vi "Open SubPanel.vi"() -> ()   [LabVIEW 2021]
panel:
  out "error out":errorcluster
  in  "error in":errorcluster
  in  "Stop Button":bool
  in  "Select VI":i32(ring) items=["Show Time", "Random Numbers", "Sine Wave"]
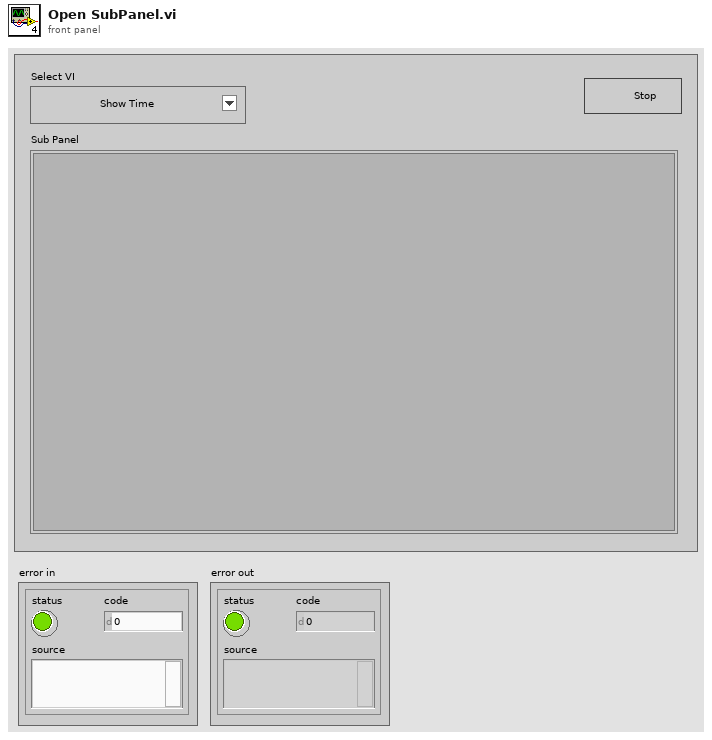
[diagram p1: front panel]
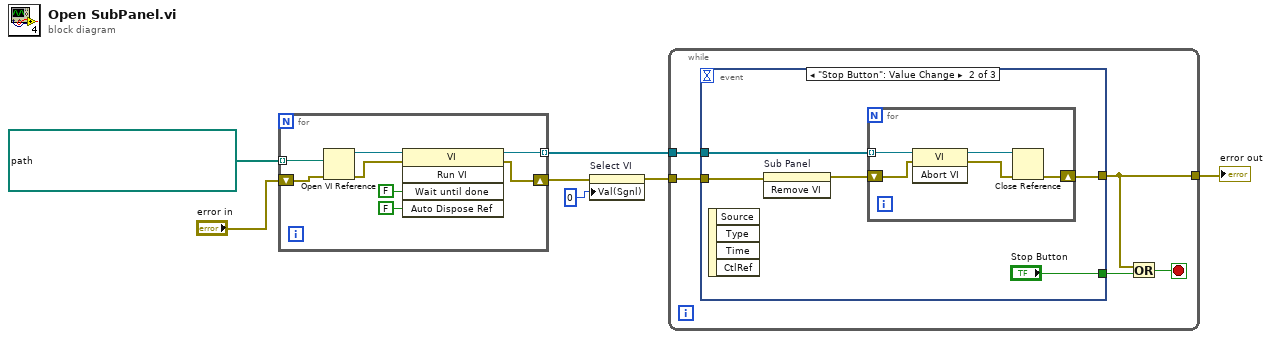
[diagram p0: block diagram]
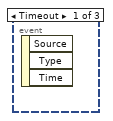
[diagram p2: hidden frame]
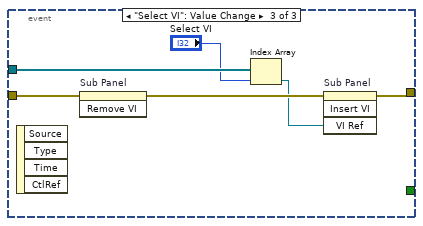
[diagram p3: hidden frame]
diagram:
  n1 = for {
    tunnel: path[] [path "F:/AGH - Inżynieria Biomedyczna (I i II stopień)/PRACA MAGISTERSKA/LABVIEW - examples (CODE)/Using SubPanels/Demo - Current Time.vi", path "F:/AGH - Inżynieria Biomedyczna (I i II stopień)/PRACA MAGISTERSKA/LABVIEW - examples (CODE)/Using SubPanels/Demo - Random Data Chart.vi", path "F:/AGH - Inżynieria Biomedyczna (I i II stopień)/PRACA MAGISTERSKA/LABVIEW - examples (CODE)/Using SubPanels/Demo - Sine Graph.vi"] -> [w15] mode=indexing
    shift-right: [w9] -> w4
    shift-left: "error in" -> [w14]
    tunnel: [w8] -> w5 mode=indexing
    n2 = Open VI Reference(vi path=w15, error in (no error)=w14) -> (vi reference=w11:refnum<vi>, error out=w10:errorcluster)  [unwired: 4 in]
    n3 = invoke class="VI" method="Run VI"(reference=w11, error in=w10, "Wait until done"=FALSE ("Wait Until Done"), "Auto Dispose Ref"=FALSE ("Auto Dispose Reference")) -> (reference out=w8:refnum<vi>, error out=w9:errorcluster)  [unwired: 1 in, 3 out]
  }
  n4 = property on="Select VI" class="Ring (strict)"(error in=w4, "Val(Sgnl)"=0 ("Value (Signaling)")) -> (error out=w3:errorcluster)  [unwired: 1 in, 1 out]
  n5 = while {
    tunnel: w5 -> [w20]
    tunnel: w3 -> [w17]
    tunnel: [w16] -> w1
    stop <- w18 stop-if-true
    n6 = event shown="[1] \"Stop Button\": Value Change" {
      selector: _ -> [_ _ _]
      dyn-events: _ -> [_ _ _]
      timeout: _ -> [_ _ _]
      tunnel: w20 -> [_ w23 w33]
      tunnel: [_ "Stop Button" _] -> w19
      tunnel: w17 -> [_ w24 w36]
      tunnel: [_ w22 w34] -> w16
      event Timeout {
        n7 = event-data() -> ()  [unwired: 1 in, 3 out]
      }
      event "Stop Button": Value Change {
        n8 = event-data() -> ()  [unwired: 1 in, 4 out]
        n9 = invoke on="Sub Panel" class="SubPnl" method="Remove VI"(error in=w24) -> (error out=w21:errorcluster)  [unwired: 2 in, 2 out]
        n10 = for {
          tunnel: w23 -> [w30] mode=indexing
          shift-right: [w26] -> w22
          shift-left: w21 -> [w29]
          n11 = invoke class="VI" method="Abort VI"(reference=w30, error in=w29) -> (reference out=w28:refnum<vi>, error out=w27:errorcluster)  [unwired: 1 in, 1 out]
          n12 = Close Reference(reference=w28, error in (no error)=w27) -> (error out=w26:errorcluster)
        }
      }
      event "Select VI": Value Change {
        n13 = event-data() -> ()  [unwired: 1 in, 4 out]
        n14 = invoke on="Sub Panel" class="SubPnl" method="Remove VI"(error in=w36) -> (error out=w35:errorcluster)  [unwired: 2 in, 2 out]
        n15 = Index Array(array=w33, index="Select VI") -> (element=w31:refnum<vi>)
        n16 = invoke on="Sub Panel" class="SubPnl" method="Insert VI"(error in=w35, "VI Ref"=w31) -> (error out=w34:errorcluster)  [unwired: 2 in, 3 out]
      }
    }
    n17 = Or(x=w16, y=w19) -> (x .or. y?=w18:bool)
  }
  "error out" <- w1
